vi "read-write config ini ring data.vi"(7 "Function":enum16{"Read", "Write"}(ring), 8 "error in (no error)":errorcluster, 10 "user data in":T1={"option data"=[]}, 11 "file name":string) -> (0 "error out":errorcluster, 2 "user data out":T1)   [LabVIEW 2024]
doc: "This VI saves (Write) and retrieves (Read) data from a configuration .ini file, regardless of the number of sectors and the keys in each sector."
uses:
  controls/ring data.ctl
  <vilib>/Utility/config.llb/Read Key (String).vi
  <vilib>/Utility/config.llb/Write Key (String).vi
  <vilib>/Utility/config.llb/NI_LVConfig.lvlib
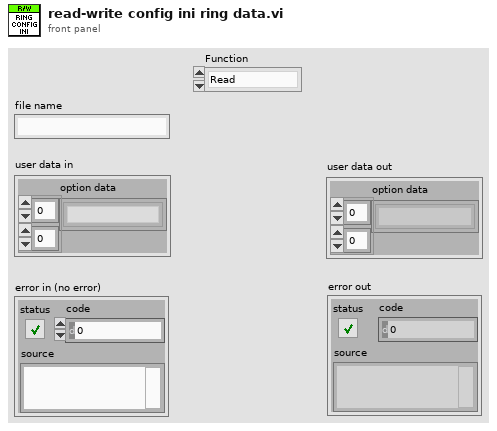
[diagram p1: front panel]
types:
  T1 = typedef "ring data.ctl" = cluster{"option data":string[][]}
  T2 = typedef "NI_LVConfig.lvlib/Config Data RefNum.ctl" = refnum<k1>
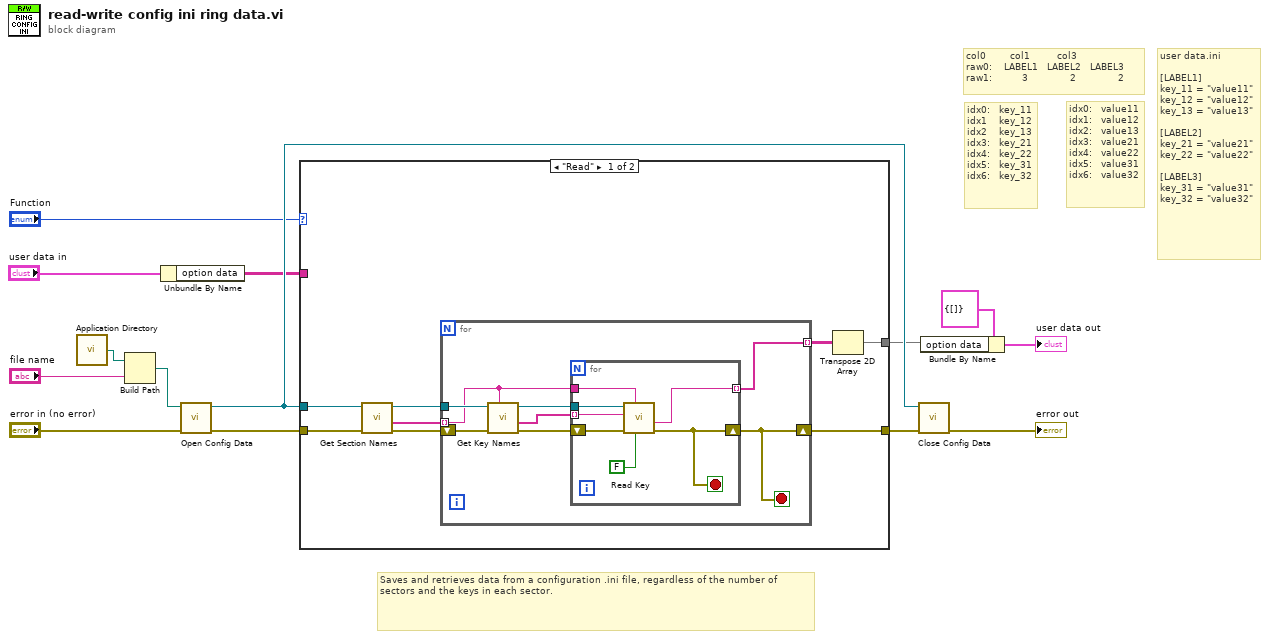
[diagram p0: block diagram]
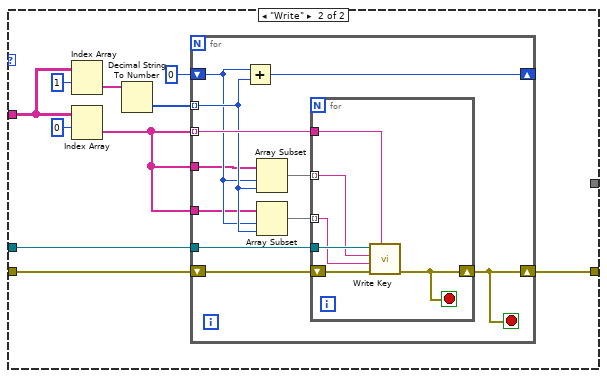
[diagram p2: hidden frame]
diagram:
  # "user data.ini\n\n[LABEL1]\nkey_11 = \"value11\"\nkey_12 = \"value12\"\nkey_13 = \"value13\"\n\n[LABEL2]\nkey_21 = \"value21\"\nkey_22 = \"value22\"\n\n[LABEL3]\nkey_31 = \"value31\"\nkey_32 = \"value32\""
  # "idx0:   value11\nidx1:   value12\nidx2:   value13\nidx3:   value21\nidx4:   value22\nidx5:   value31\nidx6:   value32"
  # "idx0:   key_11\nidx1    key_12\nidx2    key_13\nidx3:   key_21\nidx4:   key_22\nidx5:   key_31\nidx6:   key_32"
  # "col0        col1         col3   \nraw0:    LABEL1   LABEL2   LABEL3\nraw1:          3              2              2"
  # "Saves and retrieves data from a configuration .ini file, regardless of the number of sectors and the keys in each sector."
  n1 = call <vilib>:"Application Directory.vi"() -> ("Application Directory"=w10:path)
  n2 = Build Path(base path=w10, name or relative path="file name") -> (appended path=w12:path)
  n3 = Unbundle By Name("user data in") -> ("option data"=w4:string[][])
  n4 = call <vilib>:"Open Config Data.vi"("error in (no error)"="error in (no error)", "configuration file path"=w12) -> ("error out"=w14:errorcluster, "refnum"=w7:T2)  [unwired: 7 in, 1 out]
  n5 = case shown="\"Read\"" "Function" {
    tunnel: w14 -> [w20 w47]
    tunnel: [w19 w46] -> w9
    tunnel: w7 -> [w18 w45]
    tunnel: w4 -> [_ w42]
    tunnel: [w15 _] -> w1
    frame "Read" {
      n6 = call <vilib>:"Get Section Names.vi"("error in (no error)"=w20, "refnum"=w18) -> ("error out"=w21:errorcluster, "section names"=w17:string[], "refnum out"=w22:T2)  [unwired: 7 in]
      n7 = for {
        tunnel: w22 -> [w30]
        tunnel: w17 -> [w25] mode=indexing
        shift-right: [w26] -> w19
        shift-left: w21 -> [w29]
        tunnel: [w23] -> w16 mode=indexing
        stop <- w26 stop-if-true
        n8 = call <vilib>:"Get Key Names.vi"("section"=w25, "error in (no error)"=w29, "refnum"=w30) -> ("error out"=w28:errorcluster, "key names"=w24:string[], "refnum out"=w27:T2)  [unwired: 5 in, 1 out]
        n9 = for {
          shift-right: [w32] -> w26
          shift-left: w28 -> [w37]
          tunnel: w24 -> [w33] mode=indexing
          tunnel: w27 -> [w36]
          tunnel: w25 -> [w35]
          tunnel: [w34] -> w23 mode=indexing
          stop <- w32 stop-if-true
          n10 = call-poly <vilib>:"Read Key.vi"("read raw string? (F)"=FALSE, "section"=w35, "error in (no error)"=w37, "key"=w33, "refnum"=w36) -> ("error out"=w32:errorcluster, "value"=w34:string)  [unwired: 3 in, 2 out]
        }
      }
      n11 = Transpose 2D Array(2D array=w16) -> (transposed array=w15:string[][])
    }
    frame "Write" {
      n12 = Index Array(array=w42, index (row)=1) -> (element=w41:string[])  [unwired: 1 in]
      n13 = Index Array(array=w42, index (row)=0) -> (element=w38:string[])  [unwired: 1 in]
      n14 = Decimal String To Number(string=w41) -> (number=w40:i32[])  [unwired: 2 in, 1 out]
      n15 = for {
        tunnel: w45 -> [w57]
        tunnel: w38 -> [w56] mode=indexing
        shift-right: [w55] -> w46
        shift-left: w47 -> [w58]
        tunnel: w40 -> [w51] mode=indexing
        shift-right: [w53] -> _
        shift-left: 0 ("sector") -> [w50]
        tunnel: w38 -> [w49]
        tunnel: w38 -> [w48]
        stop <- w55 stop-if-true
        n16 = Add(x=w50, y=w51) -> (x+y=w53:i32)
        n17 = Array Subset(array=w49, index=w50, length=w51) -> (w54:string[])
        n18 = Array Subset(array=w48, index=w50, length=w51) -> (w52:string[])
        n19 = for {
          tunnel: w57 -> [w64]
          shift-right: [w59] -> w55
          shift-left: w58 -> [w63]
          tunnel: w56 -> [w62]
          tunnel: w54 -> [w61] mode=indexing
          tunnel: w52 -> [w60] mode=indexing
          stop <- w59 stop-if-true
          n20 = call-poly <vilib>:"Write Key.vi"("section"=w62, "error in (no error)"=w63, "value"=w60, "key"=w61, "refnum"=w64) -> ("error out"=w59:errorcluster)  [unwired: 4 in, 2 out]
        }
      }
    }
  }
  n21 = call <vilib>:"Close Config Data.vi"("error in (no error)"=w9, "refnum"=w7) -> ("error out"=→"error out":errorcluster)  [unwired: 8 in, 1 out]
  n22 = Bundle By Name(cluster=T1 {"option data"=[]} ("user data out"), "option data"=w1) -> (→"user data out":T1)
